vi "ident signals.vi"() -> ()   [LabVIEW 2015]
uses:
  <vilib>/Analysis/1siggen.llb/General Aperiodic Triangle.vi
  <vilib>/Analysis/NI_AALBase.lvlib
panel:
  out "MLS":dbl[](graph)
  out "Triangle Pattern":dbl[](graph)
  out "Gaussian WN":dbl[](graph)
  out "Uniform WN":dbl[](graph)
  out "Chirp Pattern":dbl[](graph)
  out "Sawtooth":dbl[](graph)
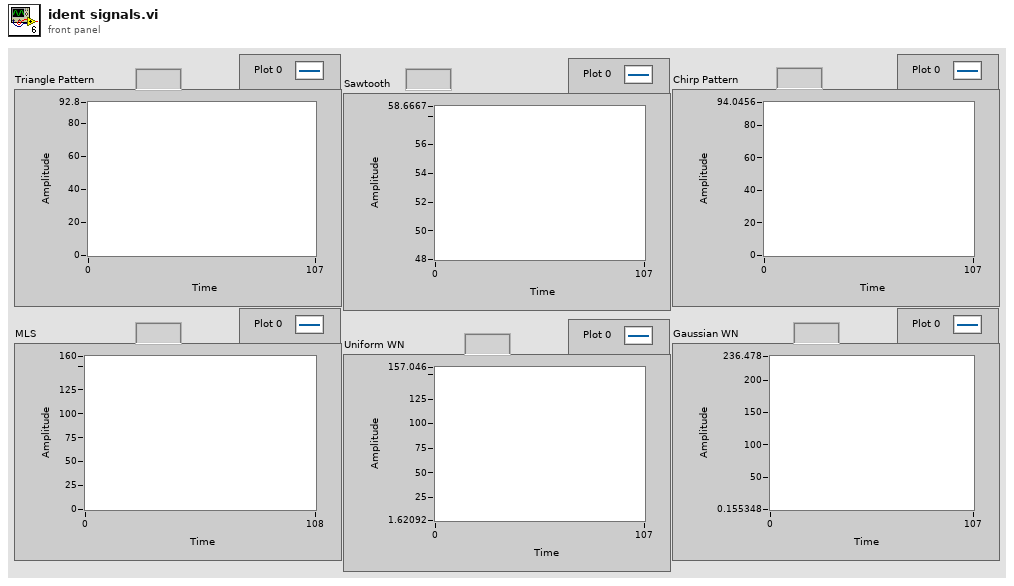
[diagram p1: front panel]
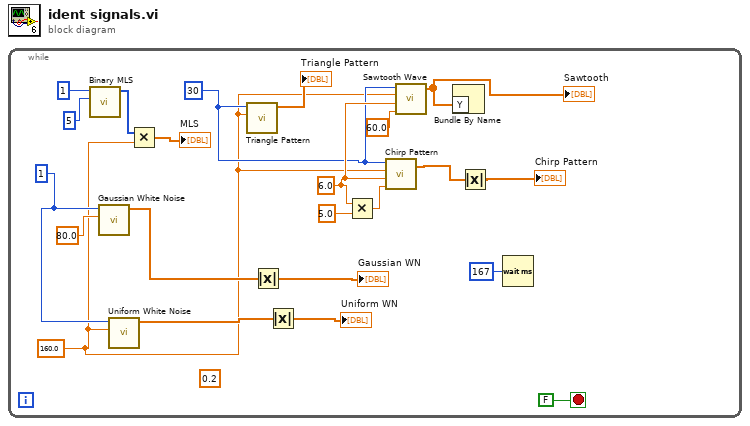
[diagram p0: block diagram]
diagram:
  n1 = while {
    stop <- FALSE stop-if-true
    w2 = 1 ("samples")
    (unwired) 0.2 ("delta t (s)")
    w19 = 6.0 ("f1")
    w1 = 160.0 ("amplitude")
    w12 = 30 ("samples")
    n2 = call <vilib>:"Binary MLS.vi"("polynomial order"=5, "samples"=i64 1) -> ("mls sequence"=w5:u8[])  [unwired: 8 in, 1 out]
    n3 = call <vilib>:"Gaussian White Noise.vi"("standard deviation"=80.0, "samples"=w2) -> ("Gaussian noise pattern"=w7:dbl[])  [unwired: 8 in, 1 out]
    n4 = call <vilib>:"Uniform White Noise.vi"("amplitude"=w1, "samples"=w2) -> ("uniform white noise"=w6:dbl[])  [unwired: 8 in, 1 out]
    n5 = Multiply(x=w5, y=w1) -> (x*y=→"MLS":dbl[])
    n6 = call <vilib>:"Triangle Pattern.vi"("amplitude"=w1, "samples"=w12) -> ("Triangle Pattern"=→"Triangle Pattern":dbl[])  [unwired: 8 in, 1 out]
    n7 = Absolute Value(x=w7) -> (abs(x)=→"Gaussian WN":dbl[])
    n8 = Absolute Value(x=w6) -> (abs(x)=→"Uniform WN":dbl[])
    n9 = Multiply(x=w19, y=5.0) -> (x*y=w14:dbl)
    n10 = call <vilib>:"Chirp Pattern.vi"("f2"=w14, "f1"=w19, "amplitude"=w1, "samples"=w12) -> ("Chirp Pattern"=w11:dbl[])  [unwired: 1 out]
    n11 = call <vilib>:"Sawtooth Wave.vi"("samples"=w12, "amplitude"=w1, "frequency"=w19, "phase in"=60.0) -> ("sawtooth wave"=w18:dbl[])  [unwired: 1 in, 2 out]
    "Sawtooth" <- w18
    n12 = Bundle By Name("Y"=w18) -> ()  [unwired: 1 in, 1 out]
    n13 = Absolute Value(x=w11) -> (abs(x)=→"Chirp Pattern":dbl[])
    n14 = Wait (ms)(milliseconds to wait=u32 167) -> ()  [unwired: 1 out]
  }
